vi "Save File Different Location During Runtime.vi"(4 "LV Program":T1=enum."DOE Stand", 6 "Number of Cycles/ File":i32=1, 7 "Debug or Inv File?":T13, 8 "error in (no error)":errorcluster, 9 "Initialize.Washer In":T4={"Appliance Details"={"FileVersionInfo"={"FileVersion"="", "ProductName"="", "InternalName"="", "CompanyName"="", "LegalCopyright"="", "FileDescription"=""}, "Dishwasher Info"={"Open Cup Weight (gm):"=0.0, "Auto Cup Weight (gm):"=0.0, "Detergent-Dish:"="", "Inlet Temperature-Dish:"="", "Cycle Mode-Dish:"="", "Unit Control-Dish:"="", "Manufacturer-Dish:"=""}, "Washer Info"={"Hot Water Temperature (Fahrenheit):"="", "Cold Water Temperature (Fahrenheit):"="", "Capacity (cu.ft):"=0.0, "Initial Cloth Weight:"=0.0, "Cloth Lot:"=0, "Model Family:"="", "Program Name:"="", "Cycle Selection:"="", "Wash Temperature:"="", "Rinse Temperature:"="", "Load Size:"=""}, "File Name Output Array"=[], "Calibration Output Array"=[], "Appliance Common"={"Engineer:"="", "Model Number:"="", "Serial Number:"="", "Comments:"="", "Station ID:"="", "Technician:"="", "TR Number:"="", "Lab ID:"="", "Voltage:"="", "Water Pressure (PSI):"="", "Test Date:"="", "Computer Name:"="", "IP Address:"="", "Ambient RH:"="", "Frequency:"="", "Build:"="", "Filename:"="", "Test Type:"="", "Load Run #:"=0, "Ambient Temperature (F):"="", "File Path:"=path "", "Cycles Per Year"=60}, "Water Heater"={"Heating Mode:"=""}, "Dryer"={"Heat Setting:"="", "Washer Water Temperature (60 ± 5°F):"=60, "Water Hardness (PPM):"=17, "Dryness Setting:"="", "Dryer Type:"="", "Exhaust:"="", "Drying Cycle:"="", "Load Type:"="", "Nominal Load Weight"="", "Dryer Initial IMC Data"={"Measured IMC (lbs)"=7.0, "Actual Initial RMC (%)"=7.0, "RMC (Desired %)"=100.0, "Bone Dry Wt(lbs)"=7.0, "Tolerance(%)"=5.0, "Actual Final RMC (%)"=0.0, "CEF (lbf/kWh)"=0.0, "Minimum Weight (lbf)"=0.0, "Average Weight (lbf)"=0.0, "Maximum Weight (lbf)"=0.0, "Measured IMC In Range?"=FALSE, "Moisture Reduction Factor"=55.5, "Field Use Factor"=1.04, "Empty Dryer Cold Weigth"=0.0, "Energy Standard"=enum."D2-Automatic Dryer", "Weight Cloth (lbs)"=0.0, "Relative Moisture Content (%)"=0.0, "Relative Moisture Content - Avg (%)"=0.0}}}, "Display Data (RLT)"={"Status Color"=0, "Serial Number Display"="", "Cycle Count Display"=0, "Station Label Display"="", "Current Run Start Time Display"=0.0, "Board ID Display"="", "RPM Display"=0, "Current Display"=0.0, "Current Path Display"=path "", "Saving Display"=FALSE, "Unit Type Display"=enum."", "Total Time On Display"=0.0, "UI Button"=FALSE}} {"Display Data (RLT)"."Current Display" format="%.2f"; "Display Data (RLT)"."Cycle Count Display" format="%04d"; "Appliance Details"."Dryer"."Dryer Initial IMC Data"."Maximum Weight (lbf)" format="%03_6g"; "Appliance Details"."Dryer"."Dryer Initial IMC Data"."Average Weight (lbf)" format="%03_6g"; "Appliance Details"."Dryer"."Dryer Initial IMC Data"."Minimum Weight (lbf)" format="%03_6g"; "Appliance Details"."Dryer"."Dryer Initial IMC Data"."CEF (lbf/kWh)" format="%03_6g"; "Appliance Details"."Dryer"."Dryer Initial IMC Data"."Actual Final RMC (%)" format="%03_6g"; "Appliance Details"."Dryer"."Dryer Initial IMC Data"."Tolerance(%)" format="%0#_6g"; "Appliance Details"."Dryer"."Dryer Initial IMC Data"."Bone Dry Wt(lbs)" format="%03_6g"; "Appliance Details"."Dryer"."Dryer Initial IMC Data"."RMC (Desired %)" format="%0#_6g"; "Appliance Details"."Dryer"."Dryer Initial IMC Data"."Actual Initial RMC (%)" format="%03_6g"; "Appliance Details"."Dryer"."Dryer Initial IMC Data"."Measured IMC (lbs)" format="%0#_6g"}, 11 "File Locations In":T2={"General Setup Paths"={"Calibration File Path"=path "", "DOE Capacity Path"=path "", "Data Folder Path"=path "", "RLT Backup Data Path"=path "", "Tool Base Path"=path "", "General Startup Config Path"=path "C:/Newfi Exe/Newfi Exe Locations.ini", "File Save Previous Run Path"=path "", "File Save Configuration Data Path"=path ""}, "Data File Paths"={"Data File Path"=path "", "Debug File Path"=path "", "Bus Log Path"=path "", "Current"=path "", "Summary"=path ""}, "New Summary Created"=FALSE, "Check Location Interval (Second)"=0}) -> (0 "error out":errorcluster, 3 "File Locations Out":T2={"General Setup Paths"={"Calibration File Path"=path "", "DOE Capacity Path"=path "", "Data Folder Path"=path "", "RLT Backup Data Path"=path "", "Tool Base Path"=path "", "General Startup Config Path"=path "C:/Newfi Exe/Newfi Exe Locations.ini", "File Save Previous Run Path"=path "", "File Save Configuration Data Path"=path ""}, "Data File Paths"={"Data File Path"=path "", "Debug File Path"=path "", "Bus Log Path"=path "", "Current"=path "", "Summary"=path ""}, "New Summary Created"=FALSE, "Check Location Interval (Second)"=0}, 5 "New File?":bool=TRUE)   [LabVIEW 2023, in "Save File.lvlib"]
uses:
  Save File.lvlib
  Type Definitions/Save File Type.ctl
  Public/Type Definitions/Save File Washer.ctl
  File Setup (Public)/Type Definition/Save File DISH Dishwasher Details.ctl
  <vilib>/Platform/fileVersionInfo.llb/FileVersionInformation.ctl
  Washer DOE/Type Definitions/DOE Appliance Common.ctl
  Custom Pallet Controls/Custom Pallet String.ctl
  File Setup (Public)/Type Definition/DPT IMC Data.ctl
  Washer DOE/Type Definitions/DOE Dryer Standard.ctl
  Public/Type Definitions/Save File Appliance Display.ctl
  Public/Type Definitions/Save File Unit Type.ctl
  File Setup (Public)/Type Definition/Save File DOE File Path Control.ctl
  File Setup (Public)/Type Definition/Save File DOE Data Save Filepaths.ctl
  File Setup (Public)/Type Definition/Save File DOE LabView Program.ctl
  File Setup.lvlib
panel:
  in  "Tab Control":enum32{"Standard Inputs", "Deubg Parameters"}(tab)=enum."Deubg Parameters"
  in  "Washer Details.TR Number:":string="14HL1234"
  in  "Serial Number":string="14HL1234"
  in  "Washer Details.Lab ID:":string="14HL1234"
  in  "Day Cycle Count":i32=25632
  in  "Debug the VI":bool
  in  "Station Label Display":string="2M1"
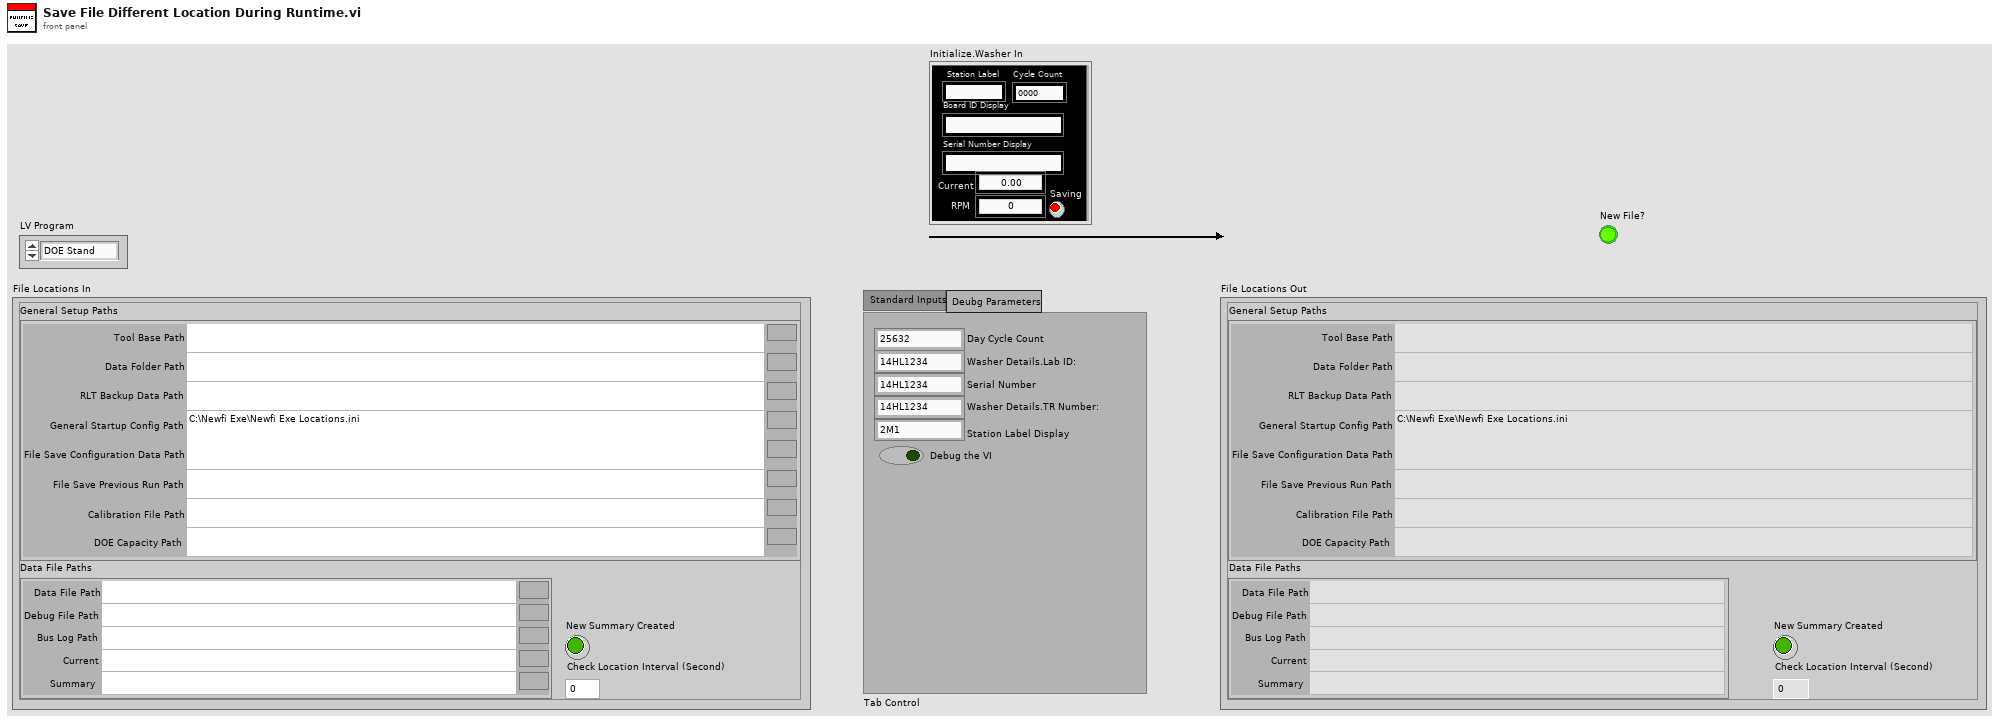
[diagram p1: front panel]
types:
  T1 = typedef "File Setup.lvlib/Save File DOE LabView Program.ctl" = enum16{"No Name Found", "DOE Stand", "Dishwasher Kitchen", "Portable Stand", "HEWH", "Dryer", "Dryer WILT", "HCC", "PRAT", "HEWH RLT", "Refrigeration", "Gas Water Heater"}
  T2 = typedef "File Setup.lvlib/Save File DOE File Path Control.ctl" = cluster{"General Setup Paths":cluster{"Calibration File Path":path, "DOE Capacity Path":path, "Data Folder Path":path, "RLT Backup Data Path":path, "Tool Base Path":path, "General Startup Config Path":path, "File Save Previous Run Path":path, "File Save Configuration Data Path":path}, "Data File Paths":T3, "New Summary Created":bool, "Check Location Interval (Second)":i32}
  T3 = typedef "File Setup.lvlib/Save File DOE Data Save Filepaths.ctl" = cluster{"Data File Path":path, "Debug File Path":path, "Bus Log Path":path, "Current":path, "Summary":path}
  T4 = typedef "Save File.lvlib/Save File Washer.ctl" = cluster{"Appliance Details":T5, "Display Data (RLT)":T11}
  T5 = typedef "File Setup.lvlib/Save File DISH Dishwasher Details.ctl" = cluster{"FileVersionInfo":T6, "Dishwasher Info":cluster{"Open Cup Weight (gm):":dbl, "Auto Cup Weight (gm):":dbl, "Detergent-Dish:":string, "Inlet Temperature-Dish:":string, "Cycle Mode-Dish:":string, "Unit Control-Dish:":string, "Manufacturer-Dish:":string}, "Washer Info":cluster{"Hot Water Temperature (Fahrenheit):":string, "Cold Water Temperature (Fahrenheit):":string, "Capacity (cu.ft):":dbl, "Initial Cloth Weight:":dbl, "Cloth Lot:":i32, "Model Family:":string, "Program Name:":string, "Cycle Selection:":string, "Wash Temperature:":string, "Rinse Temperature:":string, "Load Size:":string}, "File Name Output Array":string[][], "Calibration Output Array":string[][], "Appliance Common":T7, "Water Heater":cluster{"Heating Mode:":string}, "Dryer":cluster{"Heat Setting:":T8, "Washer Water Temperature (60 ± 5°F):":u16, "Water Hardness (PPM):":u16, "Dryness Setting:":T8, "Dryer Type:":string, "Exhaust:":string, "Drying Cycle:":string, "Load Type:":string, "Nominal Load Weight":string, "Dryer Initial IMC Data":T9}}
  T6 = typedef "FileVersionInformation.ctl" = cluster{"FileVersion":string, "ProductName":string, "InternalName":string, "CompanyName":string, "LegalCopyright":string, "FileDescription":string}
  T7 = typedef "DOE Appliance Common.ctl" = cluster{"Engineer:":string, "Model Number:":string, "Serial Number:":string, "Comments:":string, "Station ID:":string, "Technician:":string, "TR Number:":string, "Lab ID:":string, "Voltage:":string, "Water Pressure (PSI):":string, "Test Date:":string, "Computer Name:":string, "IP Address:":string, "Ambient RH:":string, "Frequency:":string, "Build:":string, "Filename:":string, "Test Type:":string, "Load Run #:":i32, "Ambient Temperature (F):":string, "File Path:":path, "Cycles Per Year":u32}
  T8 = typedef "Custom Pallet String.ctl" = string
  T9 = typedef "DPT IMC Data.ctl" = cluster{"Measured IMC (lbs)":dbl, "Actual Initial RMC (%)":dbl, "RMC (Desired %)":dbl, "Bone Dry Wt(lbs)":dbl, "Tolerance(%)":dbl, "Actual Final RMC (%)":dbl, "CEF (lbf/kWh)":dbl, "Minimum Weight (lbf)":dbl, "Average Weight (lbf)":dbl, "Maximum Weight (lbf)":dbl, "Measured IMC In Range?":bool, "Moisture Reduction Factor":dbl, "Field Use Factor":dbl, "Empty Dryer Cold Weigth":dbl, "Energy Standard":T10, "Weight Cloth (lbs)":dbl, "Relative Moisture Content (%)":dbl, "Relative Moisture Content - Avg (%)":dbl}
  T10 = typedef "DOE Dryer Standard.ctl" = enum16{"D2-Automatic Dryer", "D2-Timer Dryer", "D1-Automatic Dryer", "D1-Timer Dryer", "Other"}
  T11 = typedef "Save File Appliance Display.ctl" = cluster{"Status Color":u32, "Serial Number Display":string, "Cycle Count Display":i32, "Station Label Display":string, "Current Run Start Time Display":dbl, "Board ID Display":string, "RPM Display":u32, "Current Display":dbl, "Current Path Display":path, "Saving Display":bool, "Unit Type Display":T12, "Total Time On Display":dbl, "UI Button":bool}
  T12 = typedef "Save File.lvlib/Save File Unit Type.ctl" = enum32{"", "Viper", "Hawk", "2015"}
  T13 = typedef "Save File Type.ctl" = enum16{"Debug", "Inv and MC", "Current", "Bus File"}
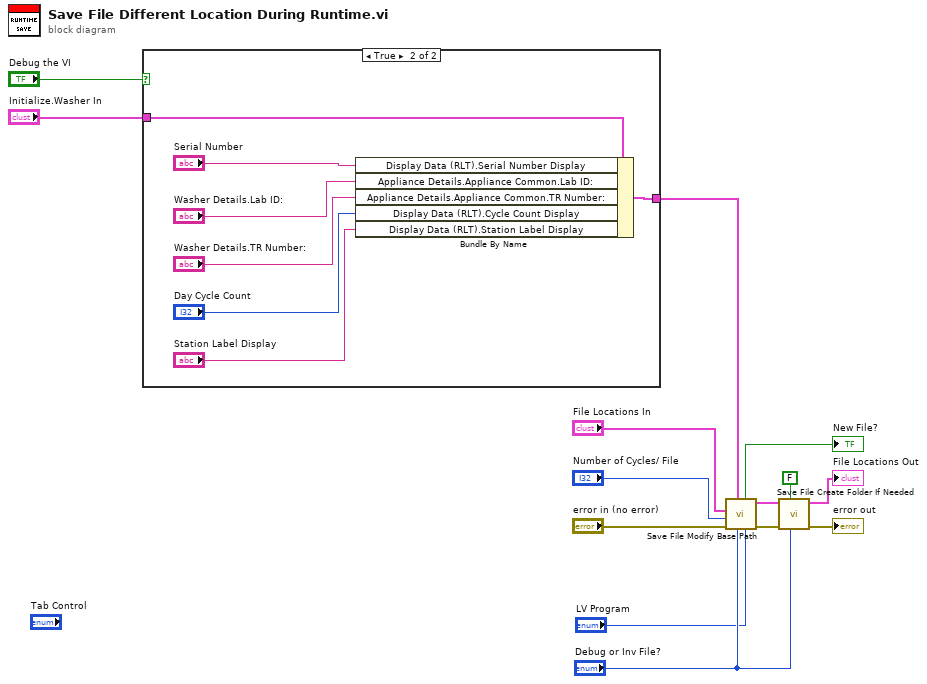
[diagram p0: block diagram]
diagram:
  n1 = case shown="True" "Debug the VI" {
    tunnel: "Initialize.Washer In" -> [w15 w22]
    tunnel: [w15 w21] -> w13
    frame False {
    }
    frame True {
      n2 = Bundle By Name(cluster=w22, "Display Data (RLT).Serial Number Display"="Serial Number", "Appliance Details.Appliance Common.Lab ID:"="Washer Details.Lab ID:", "Appliance Details.Appliance Common.TR Number:"="Washer Details.TR Number:", "Display Data (RLT).Cycle Count Display"="Day Cycle Count", "Display Data (RLT).Station Label Display"="Station Label Display") -> (w21:T4)
    }
  }
  n3 = call "Save File Modify Base Path.vi"("LV Program"="LV Program", "Debug or Inv File?"="Debug or Inv File?", "Initialize.Washer In"=w13, "error in (no error)"="error in (no error)", "Number of Cycles/ File"="Number of Cycles/ File", "File Locations In"="File Locations In") -> ("error out"=w5:errorcluster, "File Locations Out"=w4:T2, "New File?"=→"New File?":bool)  [unwired: 3 in]
  n4 = call "Save File Create Folder If Needed.vi"("Debug or Inv File?"="Debug or Inv File?", "Prevent Startup File"=FALSE, "error in (no error)"=w5, "File Locations In"=w4) -> ("error out"=→"error out":errorcluster, "File Locations Out"=→"File Locations Out":T2)  [unwired: 6 in]
